vi "SetValue.vi"(0 "VI Reference In":refnum<vi>, 2 "delimiter (>>)":string=">>", 5 "Control Path":string, 9 "Value":string[][](array[string]), 11 "Error In":errorcluster) -> (4 "VI Reference Out":refnum<vi>, 15 "Error Out":errorcluster)   [LabVIEW 2016, in "Drona.lvlib" / "ControlValue.lvlib" / "StimulusTable.lvlib"]
doc: "Sets value(signaling) for the table control.\n\nThe input control name is given as a string , incase of path, use delimiters inbetween the path."
uses:
  StimulusTable.lvlib
  <vilib>/Utility/error.llb/Error Cluster From Error Code.vi
  <vilib>/ErrorRing/Error Ring.xnode
  Drona.lvlib
  Get/GetControlRef/GetControlRef.lvlib
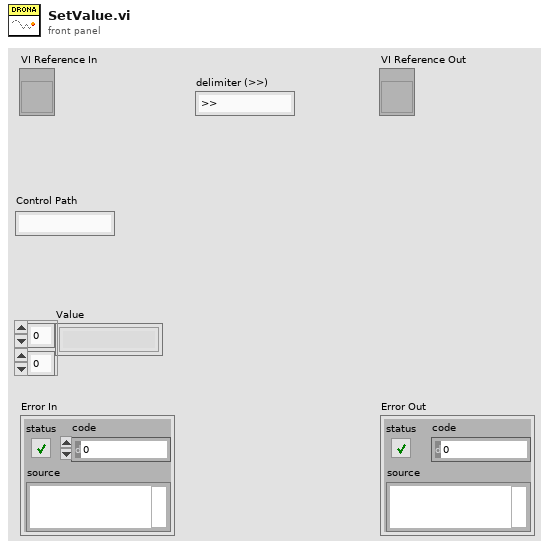
[diagram p1: front panel]
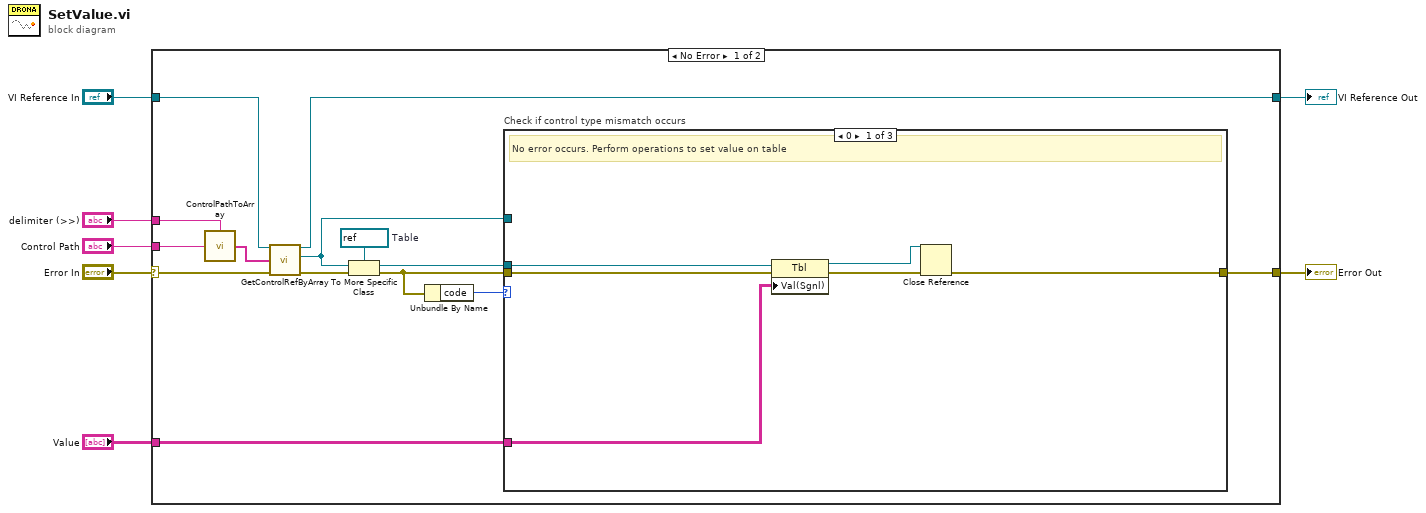
[diagram p0: block diagram]
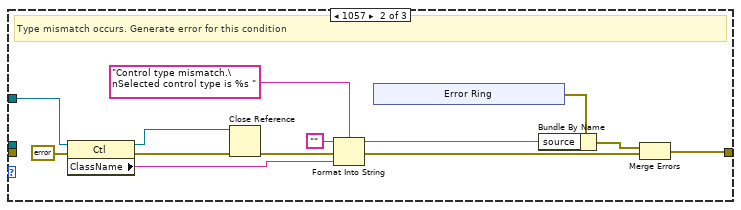
[diagram p2: hidden frame]
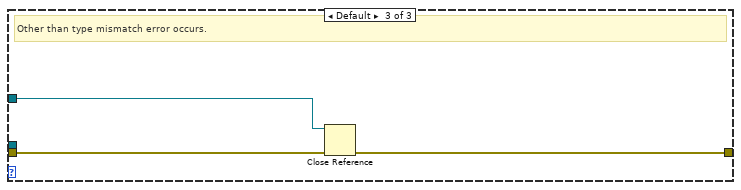
[diagram p3: hidden frame]
diagram:
  n1 = case shown="No Error" "Error In" {
    selector: "Error In" -> [w11 w50]
    tunnel: [w18 w50] -> w6
    tunnel: "VI Reference In" -> [w15 w49]
    tunnel: "Control Path" -> [w20 _]
    tunnel: [w14 w49] -> w3
    tunnel: "delimiter (>>)" -> [w19 _]
    tunnel: "Value" -> [w8 _]
    frame No Error {
      w21 = refnum<vi> refnum  # Table
      n2 = call "ControlPathToArray.vi"("Control Name"=w20, "delimiter (>>)"=w19) -> ("Control Path"=w16:string[])
      n3 = call "GetControlRefByArray.vi"("VI Reference In"=w15, "Control Path"=w16, "error In"=w11) -> ("VI Reference Out"=w14:refnum<vi>, "Ctl Refnum"=w12:refnum<vi>, "error out"=w13:errorcluster)  [unwired: 10 in]
      n4 = To More Specific Class(target class=w21, reference=w12, error in=w13) -> (specific class reference=w17:refnum<vi>, error out=w10:errorcluster)
      n5 = Unbundle By Name(w10) -> ("code"=w9:i32)
      n6 = case "Check if control type mismatch occurs" shown="0" w9 {
        tunnel: [w27 w30 w47] -> w18
        tunnel: w17 -> [w23 _ _]
        tunnel: w12 -> [_ w40 w46]
        tunnel: w10 -> [w26 _ w48]
        tunnel: w8 -> [w22 _ _]
        frame 0 {
          # "No error occurs. Perform operations to set value on table"
          n7 = property class="Tbl"(reference=w23, error in=w26, "Val(Sgnl)"=w22) -> (reference out=w24:refnum<vi>, error out=w25:errorcluster)
          n8 = Close Reference(reference=w24, error in (no error)=w25) -> (error out=w27:errorcluster)
        }
        frame 1057 {
          # "Type mismatch occurs. Generate error for this condition"
          n9 = property class="Ctl"(reference=w40, error in=errorcluster {"status"=FALSE, "code"=0, "source"=""} ("error out")) -> (reference out=w28:refnum<vi>, error out=w39:errorcluster, "ClassName"=w36:string)
          n10 = Close Reference(reference=w28, error in (no error)=w39) -> (error out=w29:errorcluster)
          n11 = Format Into String(format string="Control type mismatch.\nSelected control type is %s ", initial string="", error in=w29, w36) -> (resulting string=w33:string, error out=w31:errorcluster)
          n12 = xnode "Error Ring"() -> ("error out"=w34:errorcluster)
          n13 = Bundle By Name(cluster=w34, "source"=w33) -> (w32:errorcluster)
          n14 = Merge Errors(w32, w31) -> (w30:errorcluster)
        }
        frame Default {
          # "Other than type mismatch error occurs."
          n15 = Close Reference(reference=w46, error in (no error)=w48) -> (error out=w47:errorcluster)
        }
      }
    }
    frame Error {
    }
  }
  "Error Out" <- w6
  "VI Reference Out" <- w3
